vi "Is String Constant a State Constant.vi"(8 "error in (no error)":errorcluster, 11 "GObj Refnum":refnum<vi>) -> (0 "error out":errorcluster, 2 "Is States Constant":bool, 3 "Add States to Queue":refnum<vi>)   [LabVIEW 2013, in "JKI State Machine API.lvlib"]
uses:
  JKI State Machine API.lvlib
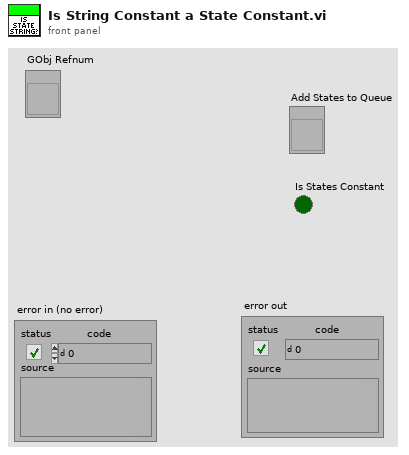
[diagram p1: front panel]
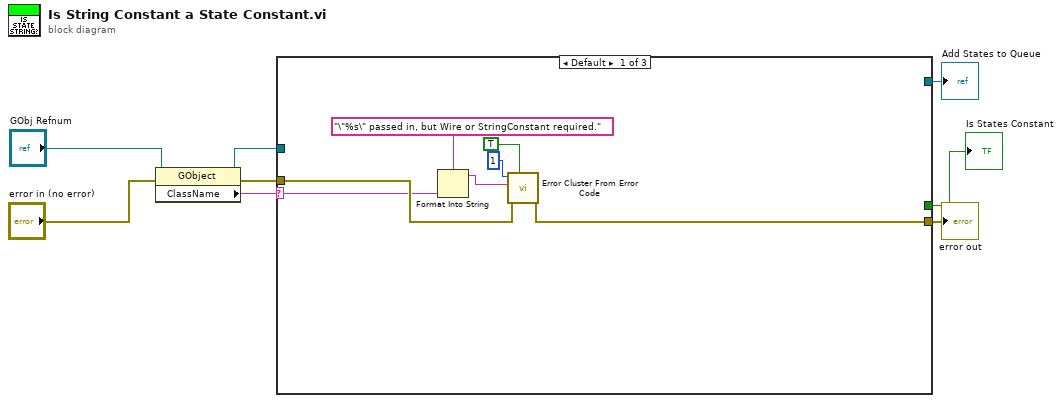
[diagram p0: block diagram]
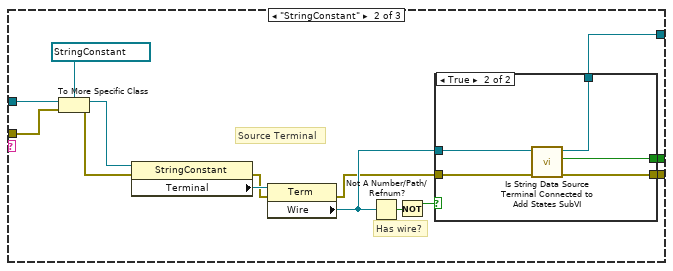
[diagram p2: hidden frame]
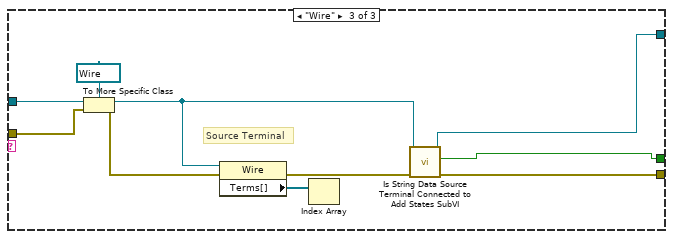
[diagram p4: hidden frame]
diagram:
  n1 = property class="GObject"(reference="GObj Refnum", error in="error in (no error)") -> (reference out=w4:refnum<vi>, error out=w2:errorcluster, "ClassName"=w1:string)
  n2 = case shown="Default" w1 {
    selector: w1 -> [w13 _ _]
    tunnel: [w14 w29 w37] -> w8
    tunnel: [_ w28 w39] -> w7
    tunnel: [_ w27 w38] -> w6
    tunnel: w4 -> [_ w23 w41]
    tunnel: w2 -> [w15 w22 w40]
    frame Default {
      n3 = Format Into String(format string="\"%s\" passed in, but Wire or StringConstant required.", w13) -> (resulting string=w11:string)  [unwired: 2 in, 1 out]
      n4 = call <vilib>:"Error Cluster From Error Code.vi"("show call chain? (False)"=TRUE, "error in (no error)"=w15, "error message (\"\")"=w11, "error code (0)"=1) -> ("error out"=w14:errorcluster)  [unwired: 5 in]
    }
    frame "StringConstant" {
      # "Has wire?"
      # "Source Terminal"
      n5 = To More Specific Class(target class=refnum<vi> refnum ("StrCnst Refnum"), reference=w23, error in=w22) -> (specific class reference=w26:refnum<vi>, error out=w24:errorcluster)
      n6 = property class="StringConstant"(reference=w26, error in=w24) -> (error out=w17:errorcluster, "Terminal"=w21:refnum<vi>)  [unwired: 1 out]
      n7 = property class="Term"(reference=w21, error in=w17) -> (error out=w16:errorcluster, "Wire"=w18:refnum<vi>)  [unwired: 1 out]
      n8 = Not A Number/Path/Refnum?(number/path/refnum=w18) -> (NaN/Path/Refnum?=w20:bool)
      n9 = Not(x=w20) -> (.not. x?=w19:bool)
      n10 = case shown="True" w19 {
        tunnel: [w30 w35] -> w29
        tunnel: [_ w34] -> w28
        tunnel: w16 -> [w30 w33]
        tunnel: [_ w32] -> w27
        tunnel: w18 -> [_ w31]
        frame False {
        }
        frame True {
          n11 = call "Is String Data Source Terminal Connected to Add States SubVI.vi"("error in (no error)"=w33, "Wire"=w31) -> ("error out"=w35:errorcluster, "Connected to Add States?"=w34:bool, "Add States SubVI"=w32:refnum<vi>)  [unwired: 6 in, 1 out]
        }
      }
    }
    frame "Wire" {
      # "Source Terminal"
      n12 = To More Specific Class(target class=refnum<vi> refnum ("Wire Refnum"), reference=w41, error in=w40) -> (specific class reference=w36:refnum<vi>, error out=w42:errorcluster)
      n13 = property class="Wire"(reference=w36, error in=w42) -> (error out=w44:errorcluster, "Terms[]"=w45:refnum<vi>[])  [unwired: 1 out]
      n14 = Index Array(array=w45) -> ()  [unwired: 1 in, 1 out]
      n15 = call "Is String Data Source Terminal Connected to Add States SubVI.vi"("error in (no error)"=w44, "Wire"=w36) -> ("error out"=w37:errorcluster, "Connected to Add States?"=w39:bool, "Add States SubVI"=w38:refnum<vi>)  [unwired: 6 in, 1 out]
    }
  }
  "error out" <- w8
  "Is States Constant" <- w7
  "Add States to Queue" <- w6
